vi "Capacitance_IS_Measure.vi"(6 "DCPower Pin":T1, 7 "Data Id":string, 8 "SCOPE Pins":T1[](array[typedef]), 9 "FGEN Pin":T1, 10 "FGEN Parameters":T2 {"Trigger Mode" items=["Single", "Continuous", "Stepped", "Burst"]}, 11 "Semiconductor Module Context":T4) -> (0 "error out":errorcluster)   [LabVIEW 2023, in "Capacitance.lvlib"]
doc: "Apply DC Bias and generate Chirp signal using FGEN.\nThe SCOPE acquires 2 channels per site and performs FFT, storing results in Site Data variable"
uses:
  Capacitance.lvlib
  <vilib>/NI_TestStand_SemiconductorModule/NI_TestStand_Semiconductor_Module.lvlibp/PinMap/General/SemiconductorModuleContext.ctl
  <vilib>/NI_TestStand_SemiconductorModule/NI_TestStand_Semiconductor_Module.lvlibp/PinMap/TagProvider/TSM_Pin.ctl
  ResourceHandling/TypeDefs/RH_FGEN_Parameters.ctl
  <instrlib>/niFgen/niFgen.llb/niFgen Trigger Mode.ctl
  <vilib>/Analysis/2dsp.llb/Real FFT.vi
  <vilib>/NI_TestStand_SemiconductorModule/NI_TestStand_Semiconductor_Module.lvlibp/PinMap/DC Power/PinToNIDCPowerSessions.vi
  <vilib>/NI_TestStand_SemiconductorModule/NI_TestStand_Semiconductor_Module.lvlibp/PinMap/Scope/PinsToNISCOPESession.vi
  <vilib>/NI_TestStand_SemiconductorModule/NI_TestStand_Semiconductor_Module.lvlibp/PinMap/FGEN/PinToNIFGenSession.vi
  <instrlib>/niScope/Acquire/Fetch/niScope Multi Fetch WDT.vi
  <vilib>/NI_TestStand_SemiconductorModule/NI_TestStand_Semiconductor_Module.lvlibp
  <vilib>/Analysis/NI_AALPro.lvlib
  Resonance/Resonance.lvlib
  ResourceHandling/ResourceHandling.lvlib
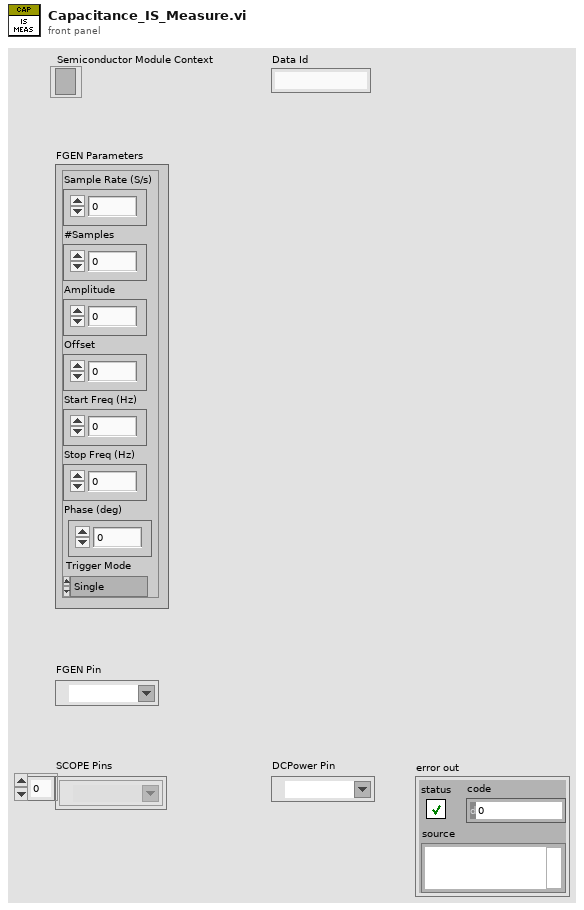
[diagram p1: front panel]
types:
  T1 = typedef "NI_TestStand_Semiconductor_Module.lvlibp/TSM_Pin.ctl" = tag
  T2 = typedef "ResourceHandling.lvlib/RH_FGEN_Parameters.ctl" = cluster{"Sample Rate (S/s)":dbl, "#Samples":i32, "Amplitude":dbl, "Offset":dbl, "Start Freq (Hz)":dbl, "Stop Freq (Hz)":dbl, "Phase (deg)":dbl, "Trigger Mode":T3}
  T3 = typedef "niFgen Trigger Mode.ctl" = i32
  T4 = typedef "NI_TestStand_Semiconductor_Module.lvlibp/SemiconductorModuleContext.ctl" = refnum<k7>
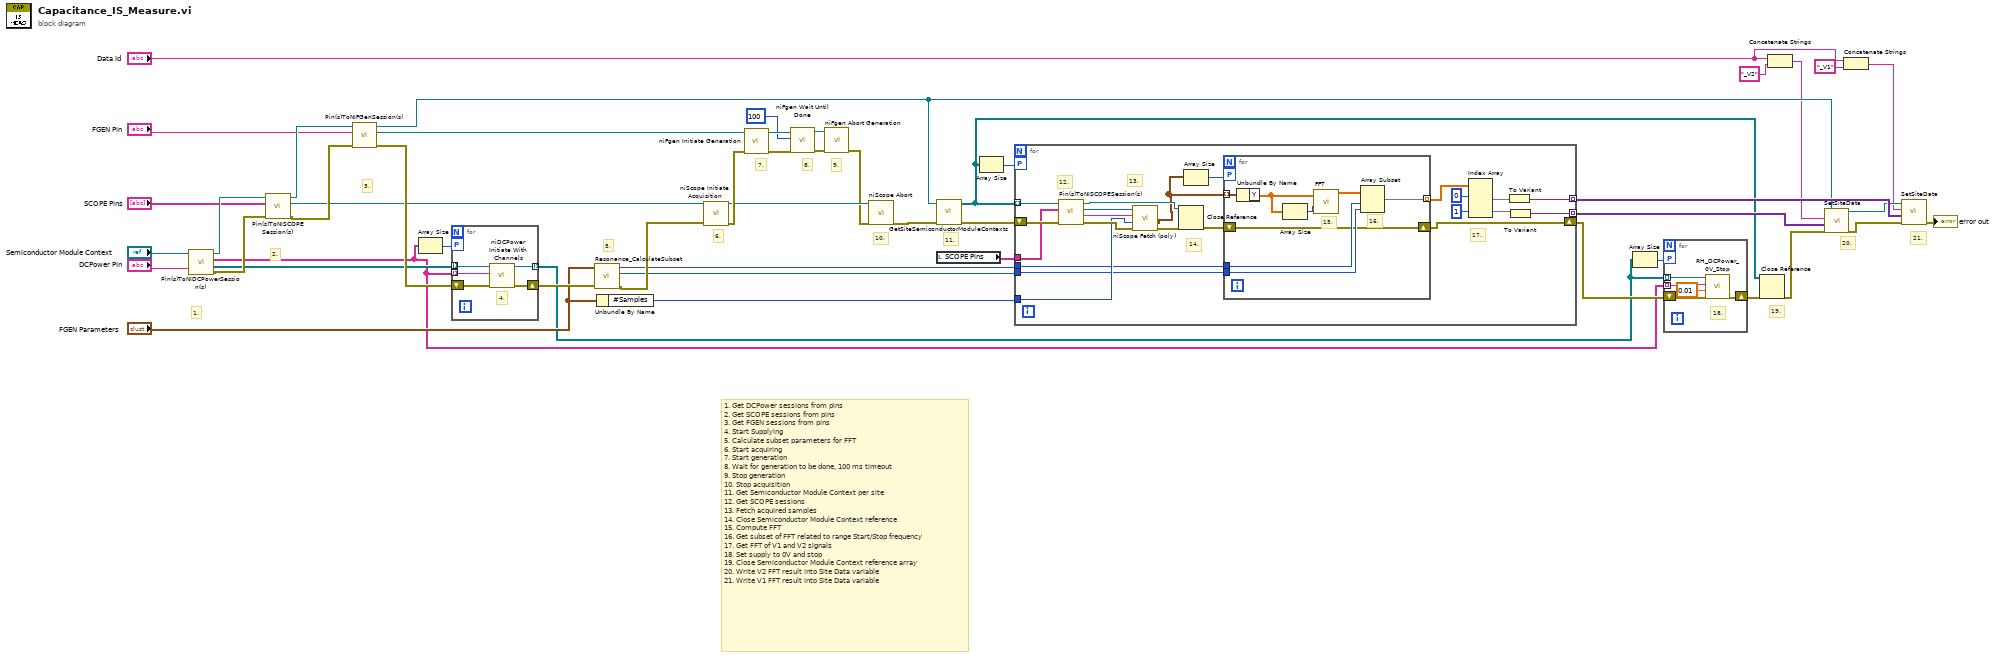
[diagram p0: block diagram]
diagram:
  # "10."
  # "9."
  # "8."
  # "7."
  # "6."
  # "1. Get DCPower sessions from pins\n2. Get SCOPE sessions from pins\n3. Get FGEN sessions from pins\n4. Start Supplying \n5. Calculate subset parameters for FFT\n6. Start acquiring\n7. Start generation\n8. Wait for generation to be done, 100 ms timeout\n9. Stop generation\n10. Stop acquisition\n11. Get Semiconductor Module Context per site\n12. Get SCOPE sessions\n13. Fetch acquired samples\n14. Close Semiconductor Module Context reference\n15. Compute FFT\n16. Get subset of FFT related to range Start/Stop frequency\n17. Get FFT of V1 and V2 signals\n18. Set supply to 0V and stop\n19. Close Semiconductor Module Context reference array\n20. Write V2 FFT result into Site Data variable\n21. Write V1 FFT result into Site Data variable"
  # "19."
  # "21."
  # "20."
  # "11."
  # "5."
  # "3."
  # "2."
  # "1."
  n1 = call-poly <vilib>:"Pin(s)ToNIDCPowerSession(s).vi"("Pin"="DCPower Pin", "Semiconductor Module Context"="Semiconductor Module Context") -> ("error out"=w47:errorcluster, "Instrument Sessions"=w42:refnum<k15>[], "Channel Strings"=w3:string[], "Semiconductor Module Context Out"=w48:T4)  [unwired: 5 in, 1 out]
  n2 = call-poly <vilib>:"Pin(s)ToNISCOPESession(s).vi"("error in (no error)"=w47, "Pins"="SCOPE Pins", "Semiconductor Module Context"=w48) -> ("error out"=w46:errorcluster, "Instrument Session"=w41:refnum<k15>, "Semiconductor Module Context Out"=w45:T4)  [unwired: 4 in, 2 out]
  n3 = call-poly <vilib>:"Pin(s)ToNIFGenSession(s).vi"("error in (no error)"=w46, "Pin"="FGEN Pin", "Semiconductor Module Context"=w45) -> ("error out"=w43:errorcluster, "Instrument Session"=w40:refnum<k15>, "Semiconductor Module Context Out"=w26:T4)  [unwired: 4 in, 2 out]
  n4 = Array Size(array=w3) -> (size(s)=w4:i32)
  n5 = for {
    shift-right: [w51] -> w36
    shift-left: w43 -> [w54]
    tunnel: w42 -> [w52] mode=indexing
    tunnel: w3 -> [w53] mode=indexing
    tunnel: [w50] -> w1 mode=indexing
    workers-P: w4 -> [_]
    # "4."
    n6 = call <instrlib>:"niDCPower Initiate With Channels.vi"("error in (no error)"=w54, "channel name"=w53, "instrument handle"=w52) -> ("error out"=w51:errorcluster, "instrument handle out"=w50:refnum<k15>)  [unwired: 7 in]
  }
  n7 = call "Resonance_CalculateSubset.vi"("error in"=w36, "FGEN Parameters"="FGEN Parameters") -> ("error out"=w35:errorcluster, "Length"=w33:i32, "Index"=w34:i32)  [unwired: 5 in, 2 out]
  n8 = Unbundle By Name("FGEN Parameters") -> ("#Samples"=w31:i32)
  n9 = call <instrlib>:"niScope Initiate Acquisition.vi"("instrument handle"=w41, "error in"=w35) -> ("instrument handle out"=w6:refnum<k15>, "error out"=w12:errorcluster)  [unwired: 12 in]
  n10 = call <instrlib>:"niFgen Initiate Generation.vi"("error in (no error)"=w12, "Instrument Handle"=w40) -> ("error out"=w10:errorcluster, "Instrument Handle Out"=w11:refnum<k15>)  [unwired: 8 in]
  n11 = call <instrlib>:"niFgen Wait Until Done.vi"("error in (no error)"=w10, "MaxTime (msec)"=100, "Instrument Handle"=w11) -> ("error out"=w7:errorcluster, "Instrument Handle Out"=w8:refnum<k15>)  [unwired: 7 in]
  n12 = call <instrlib>:"niFgen Abort Generation.vi"("error in (no error)"=w7, "Instrument Handle"=w8) -> ("error out"=w5:errorcluster)  [unwired: 8 in, 1 out]
  n13 = call <instrlib>:"niScope Abort.vi"("instrument handle"=w6, "error in"=w5) -> ("error out"=w39:errorcluster)  [unwired: 12 in, 1 out]
  n14 = call <vilib>:"GetSiteSemiconductorModuleContexts.vi"("error in (no error)"=w39, "Semiconductor Module Context"=w26) -> ("error out"=w38:errorcluster, "Site Semiconductor Module Contexts"=w16:T4[])  [unwired: 8 in]
  n15 = local read "SCOPE Pins"() -> (w15:T1[])
  n16 = Array Size(array=w16) -> (size(s)=w37:i32)
  n17 = for {
    tunnel: w16 -> [w75] mode=indexing
    shift-right: [w65] -> w19
    shift-left: w38 -> [w76]
    workers-P: w37 -> [_]
    tunnel: w34 -> [w68]
    tunnel: w33 -> [w67]
    tunnel: w31 -> [w69]
    tunnel: [w59] -> w30 mode=indexing
    tunnel: [w58] -> w29 mode=indexing
    tunnel: w15 -> [w57]
    # "17."
    # "14."
    # "13."
    # "12."
    n18 = call-poly <vilib>:"Pin(s)ToNISCOPESession(s).vi"("error in (no error)"=w76, "Pins"=w57, "Semiconductor Module Context"=w75) -> ("error out"=w73:errorcluster, "Channel List"=w72:string, "Instrument Session"=w74:refnum<k15>, "Semiconductor Module Context Out"=w70:T4)  [unwired: 4 in, 1 out]
    n19 = call-poly <instrlib>:"niScope Fetch (poly).vi"("error in"=w73, "numSamples"=w69, "channels"=w72, "instrument handle"=w74) -> ("error out"=w71:errorcluster, "wfm"=w56:waveform(dbl)[])  [unwired: 4 in, 2 out]
    n20 = Close Reference(reference=w70, error in (no error)=w71) -> (error out=w66:errorcluster)
    n21 = Array Size(array=w56) -> (size(s)=w55:i32)
    n22 = for {
      tunnel: w56 -> [w84] mode=indexing
      tunnel: w68 -> [w80]
      tunnel: w67 -> [w79]
      shift-right: [w78] -> w65
      shift-left: w66 -> [w78]
      tunnel: [w77] -> w64 mode=indexing
      workers-P: w55 -> [_]
      # "16."
      # "15."
      n23 = Unbundle By Name(w84) -> ("Y"=w82:dbl[])
      n24 = Array Size(array=w82) -> (size(s)=w83:i32)
      n25 = call-poly <vilib>:"FFT.vi"("FFT size"=w83, "X"=w82) -> ("FFT {X}"=w81:cdb[])  [unwired: 8 in, 1 out]
      n26 = Array Subset(array=w81, index=w80, length=w79) -> (w77:cdb[])
    }
    n27 = Index Array(array=w64, index (row) #1=0 ("index (row)"), index (row) #2=1 ("index (row)")) -> (element #1=w63:cdb[], element #2=w60:cdb[])  [unwired: 2 in]
    n28 = To Variant(anything=w63) -> (Variant=w59:variant)
    n29 = To Variant(anything=w60) -> (Variant=w58:variant)
  }
  n30 = Array Size(array=w1) -> (size(s)=w2:i32)
  n31 = for {
    shift-right: [w88] -> w18
    shift-left: w19 -> [w89]
    tunnel: w1 -> [w87] mode=indexing
    tunnel: w3 -> [w86] mode=indexing
    workers-P: w2 -> [_]
    # "18."
    n32 = call "RH_DCPower_0V_Stop.vi"("error in (no error)"=w89, "Settling (s)"=0.01, "Channel List"=w86, "DCPower Session In"=w87) -> ("error out"=w88:errorcluster)  [unwired: 6 in, 1 out]
  }
  n33 = Close Reference(reference=w16, error in (no error)=w18) -> (error out=w17:errorcluster)
  n34 = Concatenate Strings("Data Id", "_V2" ("string")) -> (w20:string)
  n35 = call <vilib>:"SetSiteData.vi"("error in (no error)"=w17, "Site Data"=w29, "Data Id"=w20, "Semiconductor Module Context"=w26) -> ("error out"=w28:errorcluster, "Semiconductor Module Context Out"=w25:T4)  [unwired: 5 in]
  n36 = Concatenate Strings("Data Id", "_V1" ("string")) -> (w21:string)
  n37 = call <vilib>:"SetSiteData.vi"("error in (no error)"=w28, "Site Data"=w30, "Data Id"=w21, "Semiconductor Module Context"=w25) -> ("error out"=→"error out":errorcluster)  [unwired: 5 in, 1 out]
